vi "Set RIO INI Key.vi"(8 "error in":errorcluster, 11 "Plugin in":refnum<class "Plugin.lvclass">) -> (0 "error out":errorcluster, 3 "Plugin out":refnum<class "Plugin.lvclass">)   [LabVIEW 2024, in "FPGA Addon Engine.lvlib" / "Plugin.lvclass"]
uses:
  Plugin.lvclass
  Plugin.lvclass/Plugin.ctl
  <vilib>/Utility/config.llb/NI_LVConfig.lvlib
  <vilib>/Utility/config.llb/Write Key (I32).vi
  VS Engine Abstraction/VS Engine Interface/VS Engine Interface.lvclass
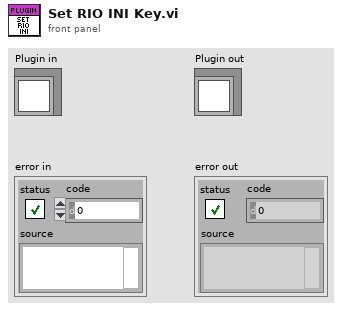
[diagram p1: front panel]
types:
  T1 = typedef "NI_LVConfig.lvlib/Config Data RefNum.ctl" = refnum<k1>
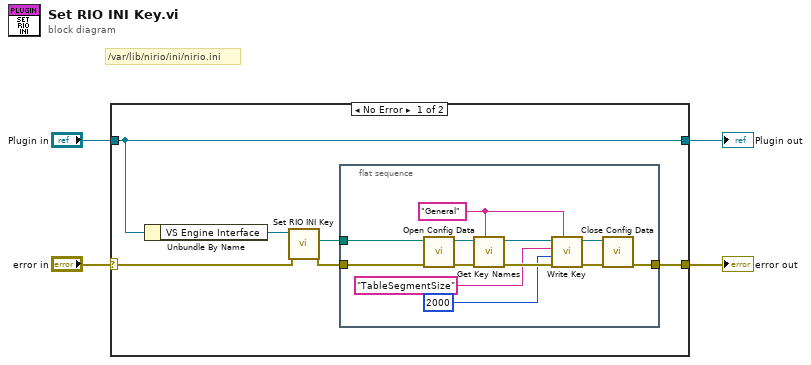
[diagram p0: block diagram]
diagram:
  # "/var/lib/nirio/ini/nirio.ini"
  n1 = case shown="No Error" "error in" {
    selector: "error in" -> [w9 w24]
    tunnel: [w10 w24] -> w3
    tunnel: "Plugin in" -> [w5 w23]
    tunnel: [w5 w23] -> w1
    frame No Error {
      n2 = Unbundle By Name(w5) -> ("VS Engine Interface"=w7:refnum<class "VS Engine Interface.lvclass">)
      n3 = call-dynamic "Set RIO INI Key.vi"("error in"=w9, "VS Engine Interface in"=w7) -> ("error out"=w8:errorcluster, "configuration file path"=w6:path)  [unwired: 7 in, 1 out]
      n4 = flat-sequence {
        tunnel: [w19] -> w10
        tunnel: w6 -> [w11]
        tunnel: w8 -> [w18]
        frame #0 {
          w15 = "General" ("section")
          n5 = call <vilib>:"Open Config Data.vi"("error in (no error)"=w18, "configuration file path"=w11) -> ("error out"=w22:errorcluster, "refnum"=w17:T1)  [unwired: 7 in, 1 out]
          n6 = call <vilib>:"Get Key Names.vi"("section"=w15, "error in (no error)"=w22, "refnum"=w17) -> ("error out"=w21:errorcluster, "refnum out"=w16:T1)  [unwired: 5 in, 2 out]
          n7 = call-poly <vilib>:"Write Key.vi"("section"=w15, "error in (no error)"=w21, "value"=2000, "key"="TableSegmentSize", "refnum"=w16) -> ("error out"=w20:errorcluster, "refnum out"=w14:T1)  [unwired: 4 in, 1 out]
          n8 = call <vilib>:"Close Config Data.vi"("error in (no error)"=w20, "refnum"=w14) -> ("error out"=w19:errorcluster)  [unwired: 8 in, 1 out]
        }
      }
    }
    frame Error {
    }
  }
  "error out" <- w3
  "Plugin out" <- w1
